vi "Main VI.vi"(11 "Error in":errorcluster) -> (15 "Error Out":errorcluster)   [LabVIEW 2020, in "Ticket Collector Lib.lvlib"]
doc: "This VI is designed to purchase tickets by inserting coins"
uses:
  Ticket Collector Lib.lvlib
  Typedef/Data Cluster.ctl
  Typedef/LCD State.ctl
  Typedef/StateMachine.ctl
  6f4c2fc5-0b10-4d86-b10f-7321068dda69.vi
  <vilib>/Comparison/Equal/Equal Functor/Equal Functor.lvclass
panel:
  in  "Coin Data":string="Bilet %s\nCena %.2f zl"
  out "Pay LED":bool
  in  "Stop":bool
  in  "Decline":bool
  in  "Pay":bool
  out "paid coins":dbl caption="ulgowy Count"
  out "Bill amount":dbl caption="normaly Count"
  out "Coin amount":string="Wrzucono"
  out "To be paid":string="Do zaplaty"
  in  "u-":bool
  in  "u+":bool
  in  "n-":bool
  in  "n+":bool
  out "Ticket2 Count":i32 caption="ulgowy Count"
  out "Ticket1 Count":i32 caption="normaly Count"
  out "LOG LCD":string
  out "Coin LCD":string
  in  "5 PLN":bool
  in  "50 Groszy":bool
  in  "2 PLN":bool
  in  "20 Groszy":bool
  in  "1 PLN":bool
  in  "10 Groszy":bool
  # "BILETOMAT"
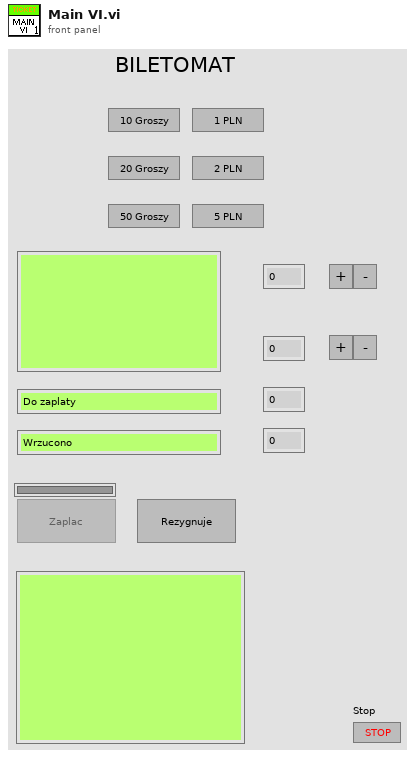
[diagram p1: front panel]
types:
  T1 = typedef "Ticket Collector Lib.lvlib/StateMachine.ctl" = enum16{"Poll", "Initialize", "InitializeUI", "InitializeLOGLCD", "ReadConfigFile", "Ticket1", "Ticket2", "CreateBeep", "MaxCoinThrown", "BuyLightUp", "Pay", "Resign", "Paid/Resigned", "CoinAdded", "FPUpdate", "Error", "Stop"}
  T2 = typedef "Ticket Collector Lib.lvlib/Data Cluster.ctl" = cluster{"Ticket prices":dbl[], "Ticket names":string[], "LCD State":T3, "LOG LCD":string, "Zaplac?":enum8{"Enabled", "Disabled", "Disabled and Grayed Out"}, "Coin LCD":string, "Ticket1 Count":i32, "Ticket2 Count":i32, "Bill amount":dbl, "Ticket1 Operator":string, "Ticket2 Operator":string, "Selected Coin Denom":string, "Amount Thrown":dbl, "Coin Count":i32[], "Coin Denom":string[], "Pay LED":bool, "Current time":timestamp}
  T3 = typedef "Ticket Collector Lib.lvlib/LCD State.ctl" = enum16{"Time", "Pay/Resign", "Default"}
  T4 = enum8{"Enabled", "Disabled", "Disabled and Grayed Out"}
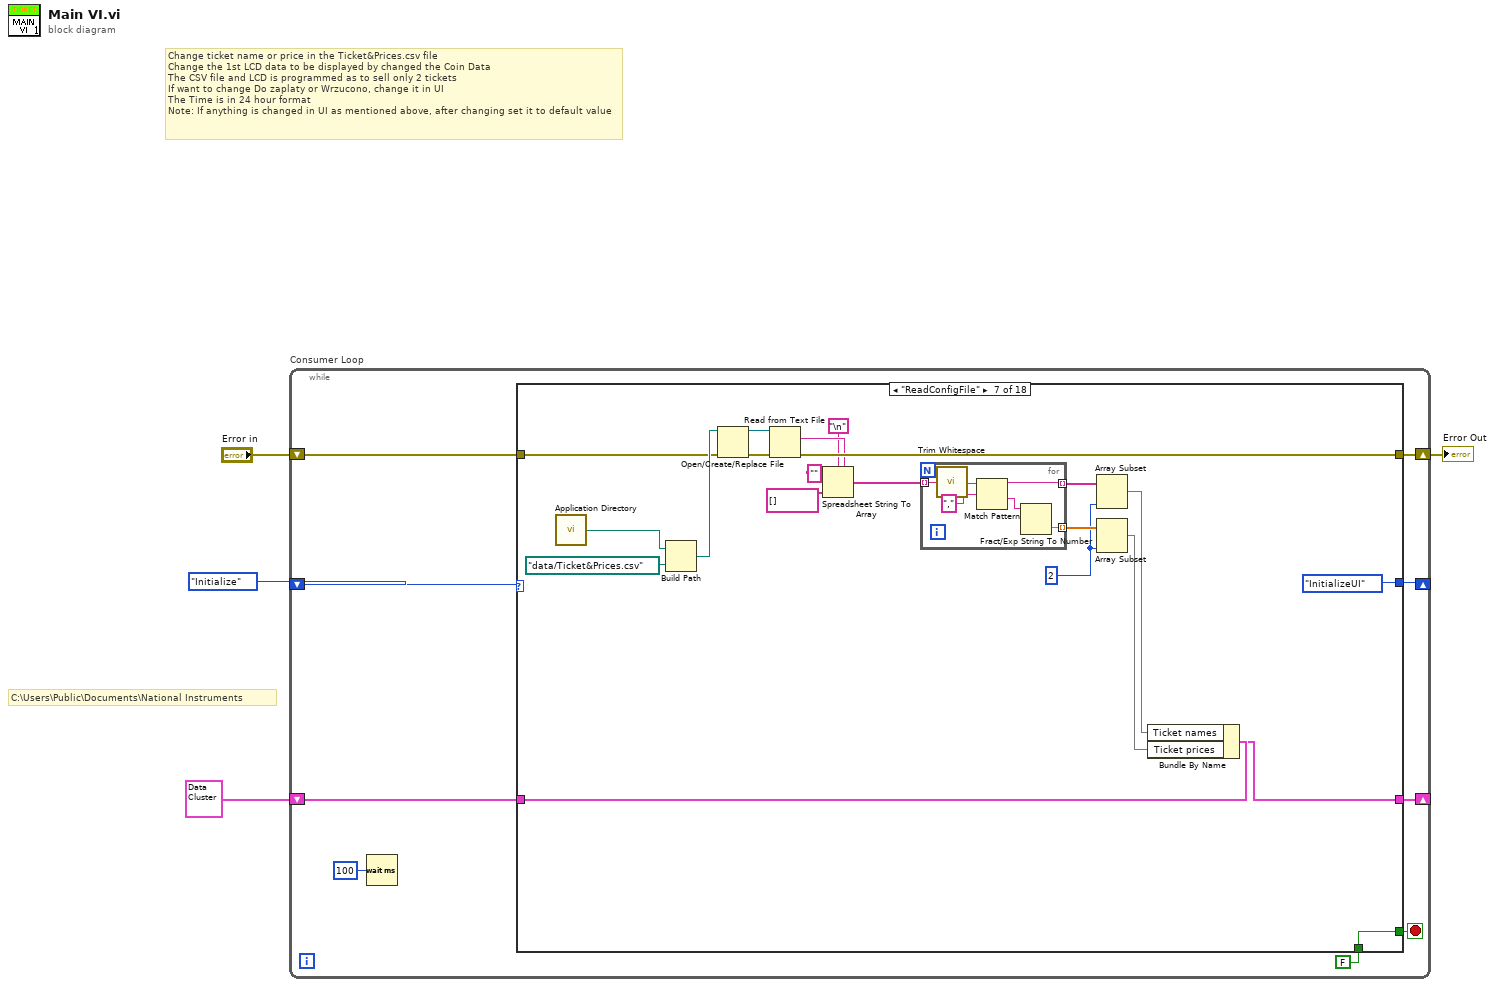
[diagram p0: block diagram]
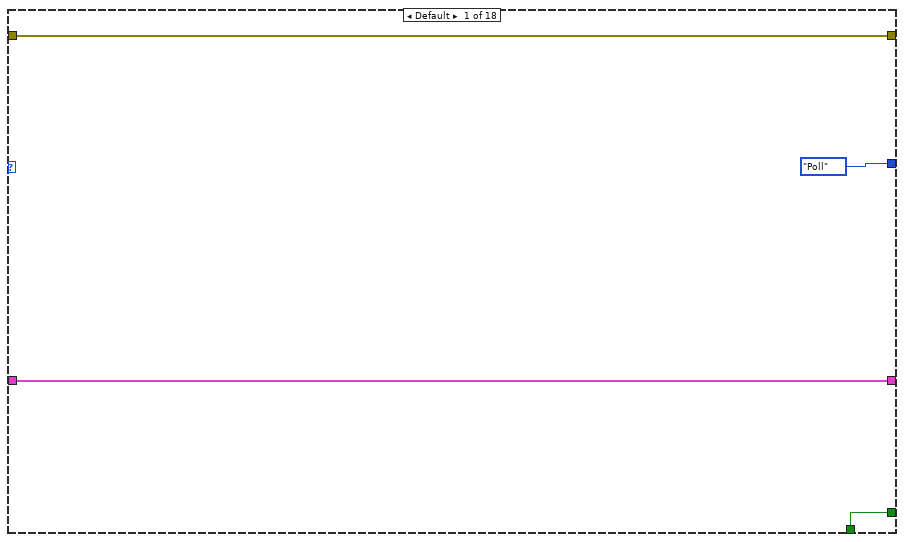
[diagram p2: hidden frame]
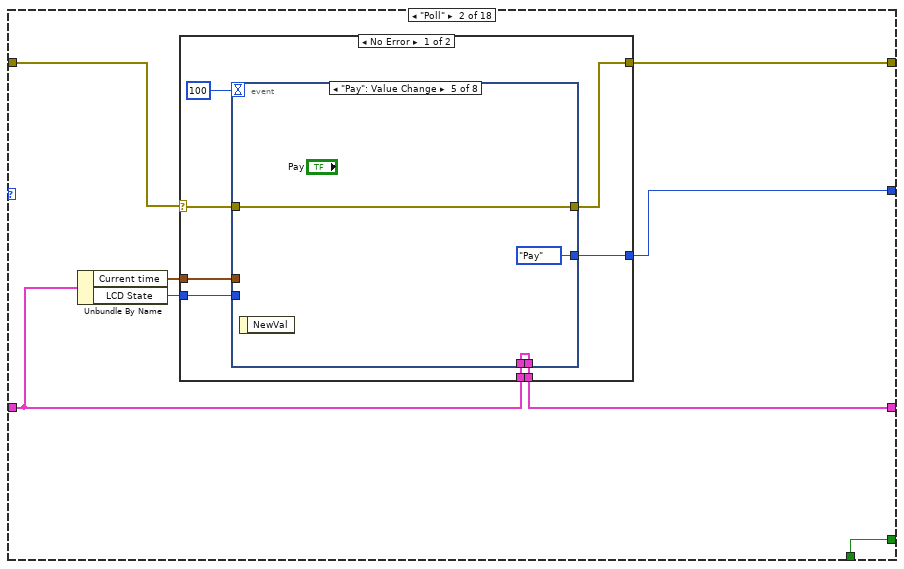
[diagram p3: hidden frame]
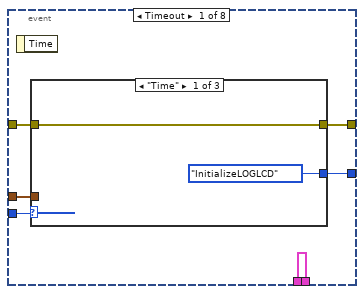
[diagram p4: hidden frame]
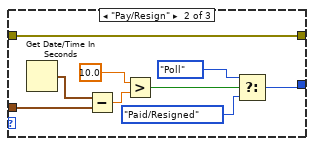
[diagram p5: hidden frame]
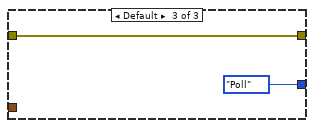
[diagram p6: hidden frame]
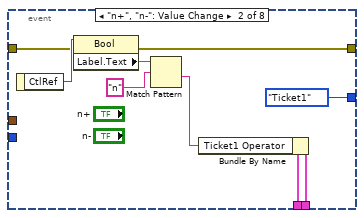
[diagram p7: hidden frame]
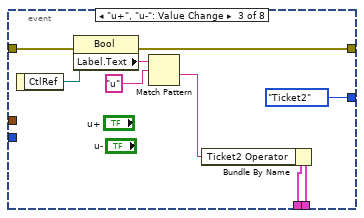
[diagram p8: hidden frame]
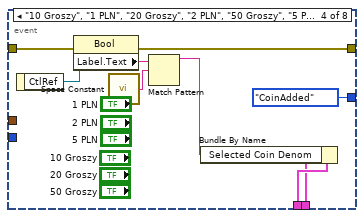
[diagram p9: hidden frame]
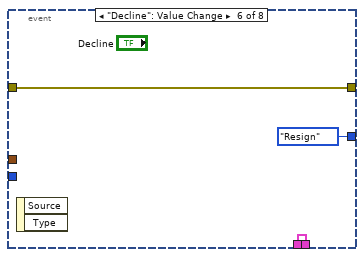
[diagram p10: hidden frame]
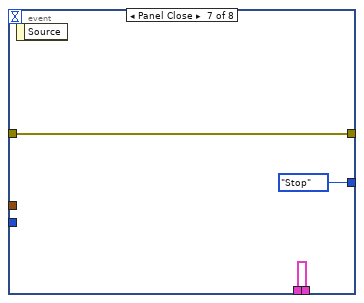
[diagram p11: hidden frame]
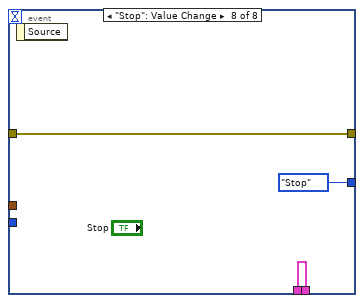
[diagram p12: hidden frame]
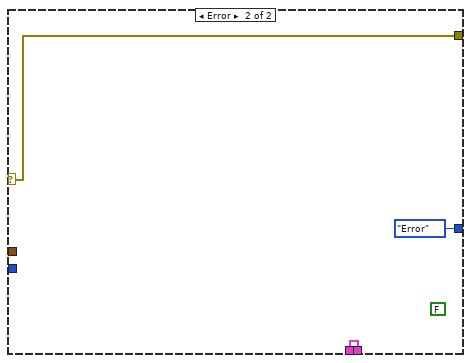
[diagram p13: hidden frame]
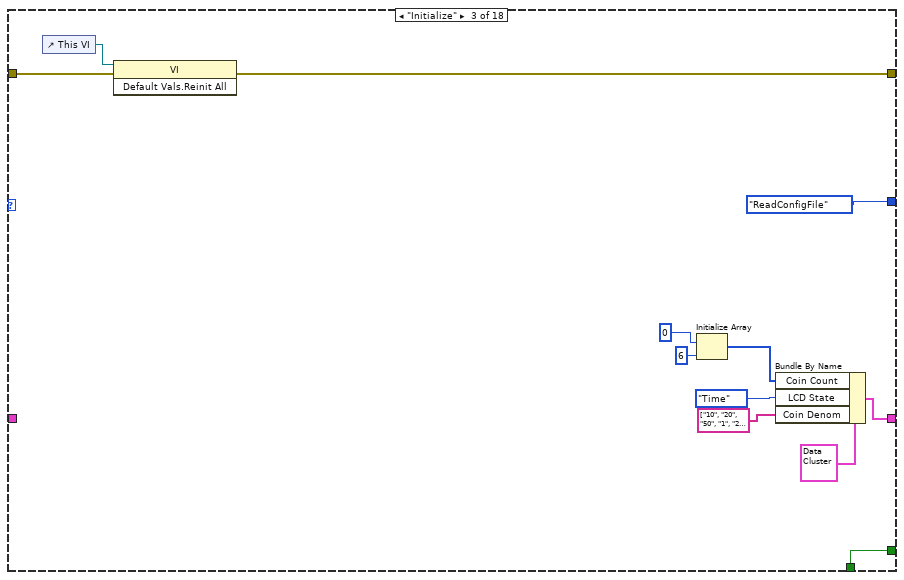
[diagram p14: hidden frame]
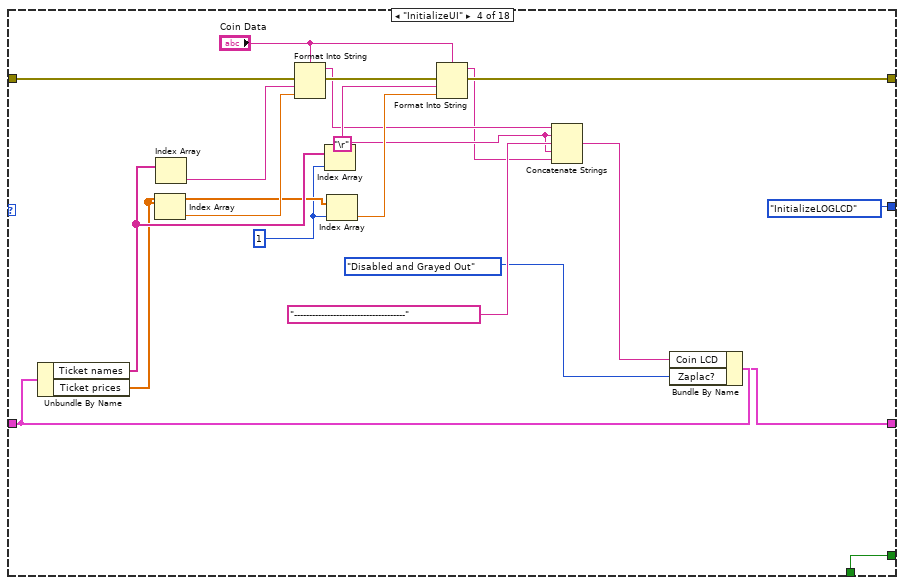
[diagram p15: hidden frame]
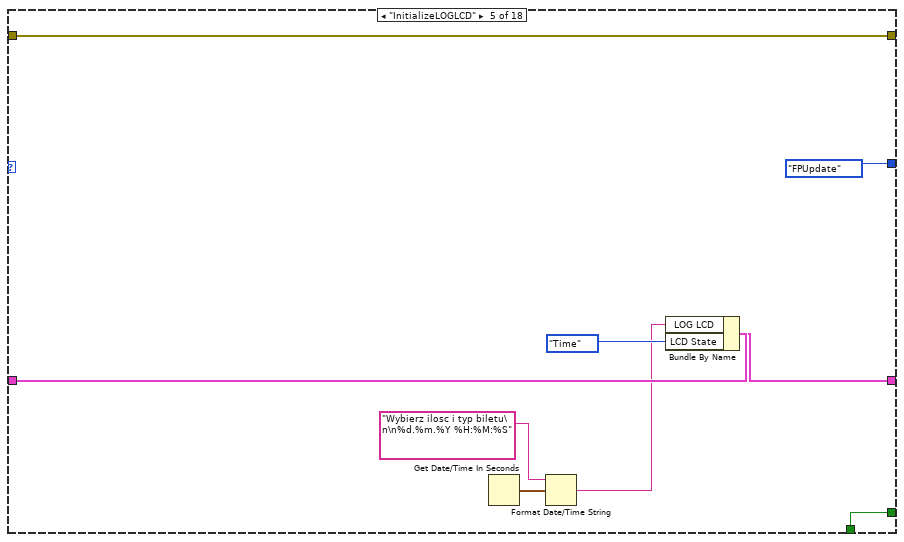
[diagram p16: hidden frame]
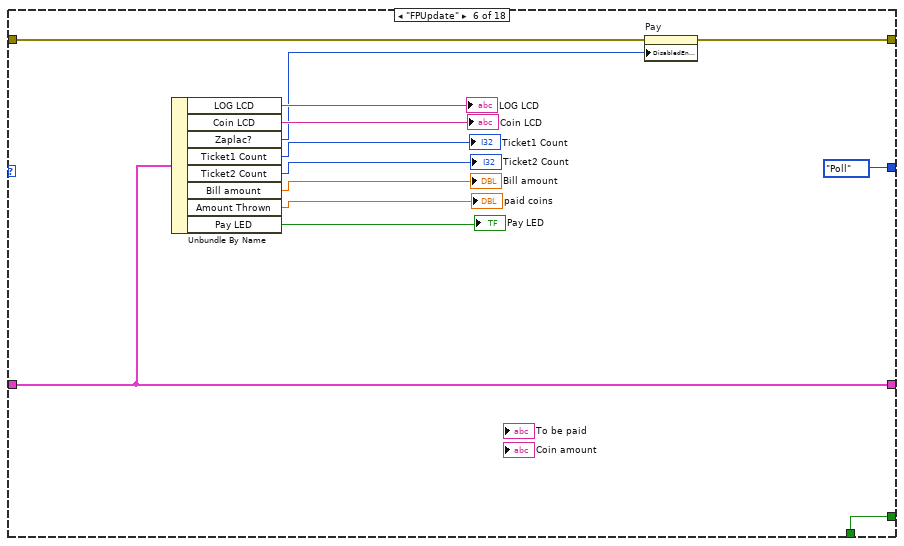
[diagram p17: hidden frame]
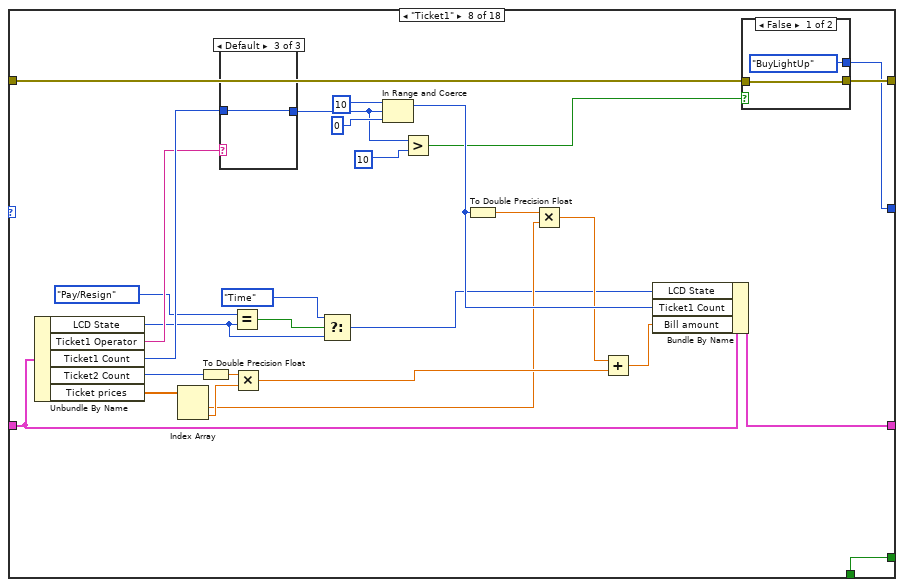
[diagram p18: hidden frame]
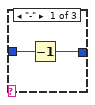
[diagram p19: hidden frame]
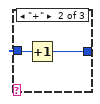
[diagram p20: hidden frame]
diagram:
  # "C:\\Users\\Public\\Documents\\National Instruments"
  # "Change ticket name or price in the Ticket&Prices.csv file\nChange the 1st LCD data to be displayed by changed the Coin Data\nThe CSV file and LCD is programmed as to sell only 2 tickets\nIf want to change Do zaplaty or Wrzucono, change it in UI\nThe Time is in 24 hour format\nNote: If anything is changed in UI as mentioned above, after changing set it to default value"
  n1 = while "Consumer Loop" {
    shift-right: [w9] -> w1
    shift-left: "Error in" -> [w13]
    shift-right: [w8] -> _
    shift-left: T2 {"Ticket prices"=[], "Ticket names"=[], "LCD State"=enum."Time", "LOG LCD"="", "Zaplac?"=enum."Enabled", "Coin LCD"="", "Ticket1 Count"=0, "Ticket2 Count"=0, "Bill amount"=0.0, "Ticket1 Operator"="", "Ticket2 Operator"="", "Selected Coin Denom"="", "Amount Thrown"=0.0, "Coin Count"=[], "Coin Denom"=["10", "20", "50", "1", "2", "5"], "Pay LED"=FALSE, "Current time"=timestamp(0 s since 1904-01-01)} ("Cluster") -> [w7]
    shift-right: [w5] -> _
    shift-left: StateMachine."Initialize" -> [w6]
    stop <- w10 stop-if-true
    n2 = Wait (ms)(milliseconds to wait=u32 100) -> ()  [unwired: 1 out]
    n3 = case shown="\"ReadConfigFile\"" w6 {
      selector: w6 -> [_ _ _ _ _ _ _ _ _ _ _ _ _ _ _ _ w356 _]
      tunnel: FALSE -> [w15 w19 w106 w127 w136 w149 w170 w204 w241 w274 w297 w304 w314 w333 w351 w355 w370 _]
      tunnel: [w15 w19 w106 w127 w136 w149 w170 w204 w241 w274 w297 w304 w314 w333 w351 w355 w370 TRUE] -> w10
      tunnel: w13 -> [w17 w22 w105 w126 w135 w145 w166 w203 w240 w271 w296 w303 w313 w328 w346 w354 w362 w378]
      tunnel: [w17 w24 w104 w117 w135 w144 w164 w185 w221 w271 w296 w303 w313 w327 w345 w354 w359 w378] -> w9
      tunnel: [w16 w20 w95 w109 w130 w148 w156 w201 w238 w272 w294 w300 w308 w331 w349 w353 w358 w377] -> w8
      tunnel: w7 -> [w16 w21 _ w111 w131 w148 w157 w202 w239 w273 w295 w301 w309 w330 w348 w353 w358 w377]
      tunnel: [StateMachine."Poll" w23 StateMachine."ReadConfigFile" StateMachine."InitializeLOGLCD" StateMachine."FPUpdate" StateMachine."Poll" StateMachine."InitializeUI" w182 w219 w263 StateMachine."BuyLightUp" StateMachine."BuyLightUp" StateMachine."FPUpdate" StateMachine."FPUpdate" StateMachine."FPUpdate" StateMachine."Initialize" w357 StateMachine."Stop"] -> w5
      frame Default {
      }
      frame "Poll" {
        n4 = Unbundle By Name(w21) -> ("Current time"=w18:timestamp, "LCD State"=w25:T3)
        n5 = case shown="No Error" w22 {
          selector: w22 -> [w29 w93]
          tunnel: w25 -> [w32 _]
          tunnel: [w31 w93] -> w24
          tunnel: [w30 StateMachine."Error"] -> w23
          tunnel: w21 -> [w28 w92]
          tunnel: [w27 w92] -> w20
          tunnel: w18 -> [w26 _]
          frame No Error {
            n6 = event shown="[4] \"Pay\": Value Change" {
              selector: _ -> [_ _ _ _ _ _ _ _]
              dyn-events: _ -> [_ _ _ _ _ _ _ _]
              timeout: 100 -> [_ _ _ _ _ _ _ _]
              tunnel: w29 -> [w39 w60 w69 w78 w82 w83 w88 w91]
              tunnel: [w37 w59 w68 w77 w82 w83 w88 w91] -> w31
              tunnel: w32 -> [w38 _ _ _ _ _ _ _]
              tunnel: [w36 StateMachine."Ticket1" StateMachine."Ticket2" StateMachine."CoinAdded" StateMachine."Pay" StateMachine."Resign" StateMachine."Stop" StateMachine."Stop"] -> w30
              tunnel: w28 -> [w35 w55 w64 w73 w80 w84 w86 w89]
              tunnel: [w35 w53 w63 w71 w80 w84 w86 w89] -> w27
              tunnel: w26 -> [w34 _ _ _ _ _ _ _]
              event Timeout {
                n7 = event-data() -> ()  [unwired: 1 in, 1 out]
                n8 = case shown="\"Time\"" w38 {
                  tunnel: w39 -> [w41 w50 w52]
                  tunnel: [w41 w50 w52] -> w37
                  tunnel: [StateMachine."InitializeLOGLCD" w43 StateMachine."Poll"] -> w36
                  tunnel: w34 -> [_ w49 _]
                  frame "Time" {
                  }
                  frame "Pay/Resign" {
                    n9 = Get Date/Time In Seconds() -> (seconds since 1Jan1904=w48:timestamp)
                    n10 = Subtract(x=w48, y=w49) -> (x-y=w47:dbl)
                    n11 = Greater?(x=10.0, y=w47) -> (0:w45:bool)
                    n12 = Select(t=StateMachine."Poll", s=w45, f=StateMachine."Paid/Resigned") -> (s? t:f=w43:T1)
                  }
                  frame Default {
                  }
                }
              }
              event "n+", "n-": Value Change {
                n13 = event-data() -> ("CtlRef"=w61:refnum<vi>)  [unwired: 1 in]
                n14 = property class="Bool"(reference=w61, error in=w60) -> (error out=w59:errorcluster, "Label.Text"=w57:string)  [unwired: 1 out]
                n15 = Match Pattern(string=w57, regular expression="n") -> (after substring=w54:string)  [unwired: 1 in, 3 out]
                n16 = Bundle By Name(cluster=w55, "Ticket1 Operator"=w54) -> (w53:T2)
              }
              event "u+", "u-": Value Change {
                n17 = event-data() -> ("CtlRef"=w70:refnum<vi>)  [unwired: 1 in]
                n18 = property class="Bool"(reference=w70, error in=w69) -> (error out=w68:errorcluster, "Label.Text"=w66:string)  [unwired: 1 out]
                n19 = Match Pattern(string=w66, regular expression="u") -> (after substring=w62:string)  [unwired: 1 in, 3 out]
                n20 = Bundle By Name(cluster=w64, "Ticket2 Operator"=w62) -> (w63:T2)
              }
              event "10 Groszy", "1 PLN", "20 Groszy", "2 PLN", "50 Groszy", "5 PLN": Value Change {
                n21 = event-data() -> ("CtlRef"=w79:refnum<vi>)  [unwired: 1 in]
                n22 = property class="Bool"(reference=w79, error in=w78) -> (error out=w77:errorcluster, "Label.Text"=w76:string)  [unwired: 1 out]
                n23 = call <vilib>:"Space Constant.vi"() -> ("String"=w75:string)
                n24 = Match Pattern(string=w76, regular expression=w75) -> (before substring=w72:string)  [unwired: 1 in, 3 out]
                n25 = Bundle By Name(cluster=w73, "Selected Coin Denom"=w72) -> (w71:T2)
              }
              event "Pay": Value Change {
                n26 = event-data() -> ()  [unwired: 1 in, 1 out]
              }
              event "Decline": Value Change {
                n27 = event-data() -> ()  [unwired: 1 in, 2 out]
              }
              event Panel Close {
                n28 = event-data() -> ()  [unwired: 1 in, 1 out]
              }
              event "Stop": Value Change {
                n29 = event-data() -> ()  [unwired: 1 in, 1 out]
              }
            }
          }
          frame Error {
            (unwired) FALSE
          }
        }
      }
      frame "Initialize" {
        n30 = control-ref of="This VI"() -> (w103:refnum<vi>)
        n31 = invoke class="VI" method="Default Vals.Reinit All"(reference=w103, error in=w105) -> (error out=w104:errorcluster)  [unwired: 1 in, 2 out]
        n32 = Initialize Array(0 ("Count"), 6 ("dimension size")) -> (w96:i32[])
        n33 = Bundle By Name(cluster=T2 {"Ticket prices"=[], "Ticket names"=[], "LCD State"=enum."Time", "LOG LCD"="", "Zaplac?"=enum."Enabled", "Coin LCD"="", "Ticket1 Count"=0, "Ticket2 Count"=0, "Bill amount"=0.0, "Ticket1 Operator"="", "Ticket2 Operator"="", "Selected Coin Denom"="", "Amount Thrown"=0.0, "Coin Count"=[], "Coin Denom"=["10", "20", "50", "1", "2", "5"], "Pay LED"=FALSE, "Current time"=timestamp(0 s since 1904-01-01)}, "Coin Count"=w96, "LCD State"=LCD_State."Time", "Coin Denom"=string[] ["10", "20", "50", "1", "2", "5"]) -> (w95:T2)
      }
      frame "InitializeUI" {
        w119 = 1 ("index")
        w113 = "\r"
        n34 = Unbundle By Name(w111) -> ("Ticket names"=w121:string[], "Ticket prices"=w120:dbl[])
        n35 = Index Array(array=w120) -> (element=w124:dbl)  [unwired: 1 in]
        n36 = Index Array(array=w121) -> (element=w125:string)  [unwired: 1 in]
        n37 = Format Into String(format string="Coin Data", error in=w126, w125, w124) -> (resulting string=w115:string, error out=w118:errorcluster)  [unwired: 1 in]
        n38 = Index Array(array=w121, index=w119) -> (element=w122:string)
        n39 = Index Array(array=w120, index=w119) -> (element=w123:dbl)
        n40 = Format Into String(format string="Coin Data", error in=w118, w122, w123) -> (resulting string=w112:string, error out=w117:errorcluster)  [unwired: 1 in]
        n41 = Concatenate Strings(w115, w113, "-------------------------------------" ("string"), w113, w112) -> (w108:string)
        n42 = Bundle By Name(cluster=w111, "Coin LCD"=w108, "Zaplac?"=T4."Disabled and Grayed Out" ("Disabled")) -> (w109:T2)
      }
      frame "InitializeLOGLCD" {
        n43 = Get Date/Time In Seconds() -> (seconds since 1Jan1904=w134:timestamp)
        n44 = Format Date/Time String(time format string (%c)="Wybierz ilosc i typ biletu\n\n%d.%m.%Y %H:%M:%S" ("format string"), seconds (now)=w134) -> (date/time string=w129:string)  [unwired: 1 in]
        n45 = Bundle By Name(cluster=w131, "LOG LCD"=w129, "LCD State"=LCD_State."Time") -> (w130:T2)
      }
      frame "FPUpdate" {
        n46 = Unbundle By Name(w148) -> ("LOG LCD"=→"LOG LCD":string, "Coin LCD"=→"Coin LCD":string, "Zaplac?"=w143:T4, "Ticket1 Count"=→"Ticket1 Count":i32, "Ticket2 Count"=→"Ticket2 Count":i32, "Bill amount"=→"Bill amount":dbl, "Amount Thrown"=→"paid coins":dbl, "Pay LED"=→"Pay LED":bool)
        n47 = property on="Pay" class="Bool"(error in=w145, "DisabledEnum"=w143) -> (error out=w144:errorcluster)  [unwired: 1 in, 1 out]
      }
      frame "ReadConfigFile" {
        w153 = 2 ("length")
        n48 = call <vilib>:"Application Directory.vi"() -> ("Application Directory"=w169:path)
        n49 = Build Path(base path=w169, name or relative path=path "data/Ticket&Prices.csv") -> (appended path=w167:path)
        n50 = Open/Create/Replace File(file path (use dialog)=w167, error in=w166) -> (refnum out=w163:refnum<file>, error out=w165:errorcluster)  [unwired: 4 in, 1 out]
        n51 = Read from Text File(file (use dialog)=w163, error in=w165) -> (text=w161:string, error out=w164:errorcluster)  [unwired: 2 in, 2 out]
        n52 = Spreadsheet String To Array(delimiter (Tab)="\n", format string="", spreadsheet string=w161, array type (2D Dbl)=string[] []) -> (array=w158:string[])
        n53 = for {
          tunnel: w158 -> [w176] mode=indexing
          tunnel: [w172] -> w155 mode=indexing
          tunnel: [w171] -> w154 mode=indexing
          n54 = call <vilib>:"Trim Whitespace.vi"("string"=w176) -> ("trimmed string"=w175:string)  [unwired: 1 in]
          n55 = Match Pattern(string=w175, regular expression=",") -> (before substring=w172:string, after substring=w173:string)  [unwired: 1 in, 2 out]
          n56 = Fract/Exp String To Number(string=w173) -> (number=w171:dbl)  [unwired: 3 in, 1 out]
        }
        n57 = Array Subset(array=w155, length=w153) -> (w152:string[])  [unwired: 1 in]
        n58 = Array Subset(array=w154, length=w153) -> (w151:dbl[])  [unwired: 1 in]
        n59 = Bundle By Name(cluster=w157, "Ticket names"=w152, "Ticket prices"=w151) -> (w156:T2)
      }
      frame "Ticket1" {
        n60 = Unbundle By Name(w202) -> ("LCD State"=w179:T3, "Ticket1 Operator"=w183:string, "Ticket1 Count"=w200:i32, "Ticket2 Count"=w195:i32, "Ticket prices"=w198:dbl[])
        n61 = Index Array(array=w198) -> (element #1=w190:dbl, element #2=w192:dbl)  [unwired: 2 in]
        n62 = To Double Precision Float(number=w195) -> (double precision float=w194:dbl)
        n63 = case shown="Default" w183 {
          tunnel: w200 -> [w205 w208 w209]
          tunnel: [w206 w207 w209] -> w184
          frame "-" {
            n64 = Decrement(x=w205) -> (x-1=w206:i32)
          }
          frame "+" {
            n65 = Increment(x=w208) -> (x+1=w207:i32)
          }
          frame Default {
          }
        }
        n66 = Equal?(x=LCD_State."Pay/Resign", y=w179) -> (x = y?=w180:bool)
        n67 = Multiply(x=w194, y=w192) -> (x*y=w197:dbl)
        n68 = Select(t=LCD_State."Time", s=w180, f=w179) -> (s? t:f=w177:T3)
        n69 = In Range and Coerce(upper limit=10, x=w184, lower limit=0) -> (coerced(x)=w193:i32)  [unwired: 1 out]
        n70 = Greater?(x=w184, y=10) -> (0:w187:bool)
        n71 = To Double Precision Float(number=w193) -> (double precision float=w191:dbl)
        n72 = Multiply(x=w191, y=w190) -> (x*y=w189:dbl)
        n73 = Add(x=w189, y=w197) -> (x+y=w196:dbl)
        n74 = Bundle By Name(cluster=w202, "LCD State"=w177, "Ticket1 Count"=w193, "Bill amount"=w196) -> (w201:T2)
        n75 = case shown="False" w187 {
          tunnel: w203 -> [w211 w213]
          tunnel: [w211 w213] -> w185
          tunnel: [StateMachine."BuyLightUp" StateMachine."CreateBeep"] -> w182
          frame False {
          }
          frame True {
          }
        }
      }
      frame "Ticket2" {
        n76 = Unbundle By Name(w239) -> ("LCD State"=w216:T3, "Ticket2 Operator"=w220:string, "Ticket2 Count"=w237:i32, "Ticket1 Count"=w231:i32, "Ticket prices"=w234:dbl[])
        n77 = Index Array(array=w234) -> (element #1=w226:dbl, element #2=w225:dbl)  [unwired: 2 in]
        n78 = To Double Precision Float(number=w231) -> (double precision float=w230:dbl)
        n79 = case shown="Default" w220 {
          tunnel: w237 -> [w242 w245 w246]
          tunnel: [w243 w244 w246] -> w224
          frame "-" {
            n80 = Decrement(x=w242) -> (x-1=w243:i32)
          }
          frame "+" {
            n81 = Increment(x=w245) -> (x+1=w244:i32)
          }
          frame Default {
          }
        }
        n82 = Multiply(x=w230, y=w226) -> (x*y=w233:dbl)
        n83 = Equal?(x=LCD_State."Pay/Resign", y=w216) -> (x = y?=w217:bool)
        n84 = Select(t=LCD_State."Time", s=w217, f=w216) -> (s? t:f=w214:T3)
        n85 = In Range and Coerce(upper limit=10, x=w224, lower limit=0) -> (coerced(x)=w229:i32)  [unwired: 1 out]
        n86 = Greater?(x=w224, y=10) -> (0:w222:bool)
        n87 = To Double Precision Float(number=w229) -> (double precision float=w228:dbl)
        n88 = Multiply(x=w228, y=w225) -> (x*y=w227:dbl)
        n89 = Add(x=w227, y=w233) -> (x+y=w232:dbl)
        n90 = Bundle By Name(cluster=w239, "Ticket2 Count"=w229, "Bill amount"=w232, "LCD State"=w214) -> (w238:T2)
        n91 = case shown="False" w222 {
          tunnel: w240 -> [w248 w250]
          tunnel: [w248 w250] -> w221
          tunnel: [StateMachine."BuyLightUp" StateMachine."CreateBeep"] -> w219
          frame False {
          }
          frame True {
          }
        }
      }
      frame "CoinAdded" {
        n92 = Unbundle By Name(w273) -> ("Coin Count"=w256:i32[], "Coin Denom"=w267:string[], "Amount Thrown"=w270:dbl, "Selected Coin Denom"=w268:string, "LCD State"=w254:T3)
        n93 = Equal?(x=LCD_State."Pay/Resign", y=w254) -> (x = y?=w252:bool)
        n94 = case shown="\"10\"" w268 {
          tunnel: [0.0 ("x") 0.1 ("x") 0.2 ("x") 0.5 ("x") 1.0 ("x") 2.0 ("x") 5.0 ("x")] -> w261
          frame Default {
          }
          frame "10" {
          }
          frame "20" {
          }
          frame "50" {
          }
          frame "1" {
          }
          frame "2" {
          }
          frame "5" {
          }
        }
        n95 = Select(t=LCD_State."Time", s=w252, f=w254) -> (s? t:f=w251:T3)
        n96 = call "Search Unsorted 1D Array.vim"("element"=w268, "unsorted 1D array"=w267) -> ("index of element"=w258:i32)  [unwired: 9 in]
        n97 = Index Array(array=w256, index=w258) -> (element=w266:i32)
        n98 = Increment(x=w266) -> (x+1=w262:i32)
        n99 = Greater?(x=w262, y=10) -> (0:w264:bool)
        n100 = case shown="False" w264 {
          tunnel: [10 ("y") w279] -> w259
          tunnel: [StateMachine."MaxCoinThrown" StateMachine."BuyLightUp"] -> w263
          tunnel: w262 -> [_ w279]
          tunnel: w261 -> [_ w278]
          tunnel: [0.0 ("x") w278] -> w260
          frame True {
          }
          frame False {
          }
        }
        n101 = Replace Array Subset(array=w256, new element=w259, index=w258) -> (w257:i32[])
        n102 = Add(x=w260, y=w270) -> (x+y=w269:dbl)
        n103 = Bundle By Name(cluster=w273, "Coin Count"=w257, "Amount Thrown"=w269, "LCD State"=w251) -> (w272:T2)
      }
      frame "CreateBeep" {
        n104 = call <vilib>:"Beep.vi"("use system alert? (T)"=FALSE, "duration (msec)"=u32 200, "frequency (Hz)"=u32 800) -> ()  [unwired: 9 in]
        n105 = Bundle By Name(cluster=w295, "LOG LCD"="Wybrano maksymalna ilosc biletów", "LCD State"=LCD_State."Default") -> (w294:T2)
      }
      frame "MaxCoinThrown" {
        n106 = Bundle By Name(cluster=w301, "LOG LCD"="Wrzucono maksymalna ilosc nominalow tego typu", "LCD State"=LCD_State."Default") -> (w300:T2)
      }
      frame "BuyLightUp" {
        n107 = Unbundle By Name(w309) -> ("Amount Thrown"=w311:dbl, "Bill amount"=w310:dbl)
        n108 = Greater?(x=w311, y=w310) -> (0:w307:bool)
        n109 = case shown="False" w307 {
          tunnel: [FALSE ("Pay LED") TRUE ("Pay LED")] -> w306
          tunnel: [T4."Disabled and Grayed Out" ("Zaplac?") T4."Enabled" ("Zaplac?")] -> w305
          frame False {
          }
          frame True {
          }
        }
        n110 = Bundle By Name(cluster=w309, "Pay LED"=w306, "Zaplac?"=w305) -> (w308:T2)
      }
      frame "Pay" {
        n111 = Unbundle By Name(w330) -> ("Ticket1 Count"=w326:i32, "Ticket2 Count"=w325:i32, "Amount Thrown"=w324:dbl, "Bill amount"=w323:dbl)
        n112 = Subtract(x=w324, y=w323) -> (x-y=w322:dbl)
        n113 = Format Into String(format string="Sprzedano :\n%d – biletow normalnych\n%d – biletow ulgowych\nReszta : %.1f" ("LOG LCD"), error in=w328, w326, w325, w322) -> (resulting string=w321:string, error out=w327:errorcluster)  [unwired: 1 in]
        n114 = Get Date/Time In Seconds() -> (seconds since 1Jan1904=w319:timestamp)
        n115 = Bundle By Name(cluster=w330, "Current time"=w319, "LCD State"=LCD_State."Pay/Resign", "LOG LCD"=w321) -> (w331:T2)
      }
      frame "Resign" {
        n116 = Unbundle By Name(w348) -> ("Amount Thrown"=w341:dbl, "Coin Count"=w340:i32[])
        n117 = Index Array(array=w340) -> (element #1=w334:i32, element #2=w335:i32, element #3=w336:i32, element #4=w337:i32, element #5=w338:i32, element #6=w339:i32)  [unwired: 6 in]
        n118 = Format Into String(format string="Reszta : %.1f\nZwrocone nominaly:\n5 PLN : %d\n2 PLN : %d\n1 PLN : %d\n50 Groszy : %d\n20 Groszy : %d\n10 Groszy : %d" ("LOG LCD"), error in=w346, w341, w339, w338, w337, w336, w335, w334) -> (resulting string=w344:string, error out=w345:errorcluster)  [unwired: 1 in]
        n119 = Get Date/Time In Seconds() -> (seconds since 1Jan1904=w342:timestamp)
        n120 = Bundle By Name(cluster=w348, "Current time"=w342, "LCD State"=LCD_State."Pay/Resign", "LOG LCD"=w344) -> (w349:T2)
      }
      frame "Paid/Resigned" {
      }
      frame "Error" {
        n121 = Unbundle By Name(w362) -> ("code"=w368:i32, "source"=w367:string)
        n122 = call <vilib>:"Clear Errors.vi"("error in (no error)"=w362, "specific error code to clear (0: all)"=w368) -> ("error out"=w369:errorcluster)  [unwired: 4 in, 1 out]
        n123 = Format Into String(format string="Error occurred at state : \"%s\"\nError code : \"%d\"\nError source : \"%s\"", error in=w369, w356, w368, w367) -> (resulting string=w363:string, error out=w360:errorcluster)  [unwired: 1 in]
        n124 = Two Button Dialog(message=w363, 1:"Exit" ("F button name (\"Cancel\")"), 2:"Continue" ("T button name (\"OK\")")) -> (T button?=w361:bool)
        n125 = case shown="True" w361 {
          tunnel: w360 -> [w372 w374]
          tunnel: [w372 w374] -> w359
          tunnel: [StateMachine."Stop" StateMachine."Stop"] -> w357
          frame True {
            # "Add Cases if needed"
          }
          frame False {
          }
        }
      }
      frame "Stop" {
      }
    }
  }
  "Error Out" <- w1
